vi "IO test DAQ read write.vi"() -> ()   [LabVIEW 2016]
panel:
  in  "Array 3":dbl[](array[numeric])
  in  "Array 2":bool[](array[boolean])
  out "Array":bool[](array[boolean])
  in  "Tab Control":enum32{"Page 1", "Page 2"}(tab)
  in  "write":bool
  in  "Read":bool
  in  "stop":bool
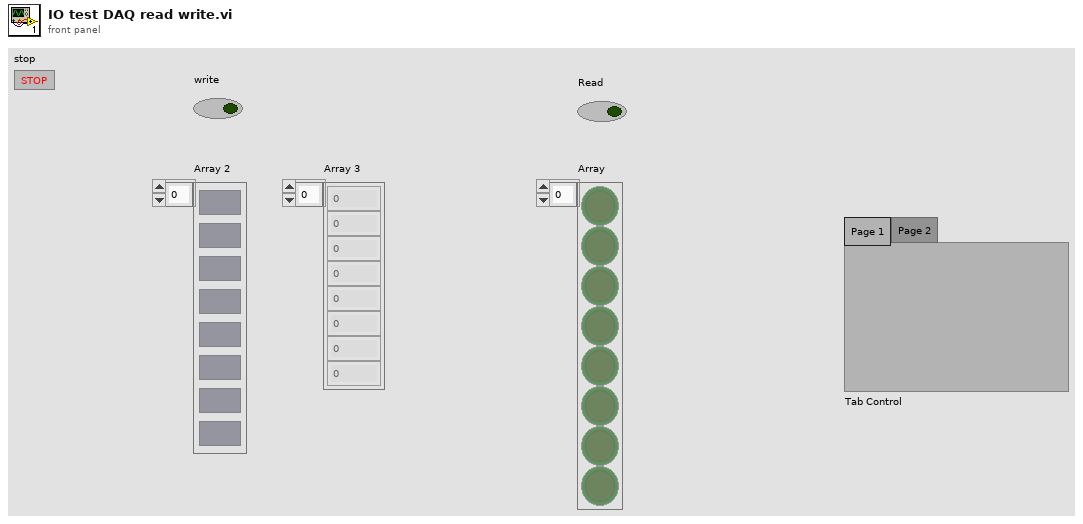
[diagram p1: front panel]
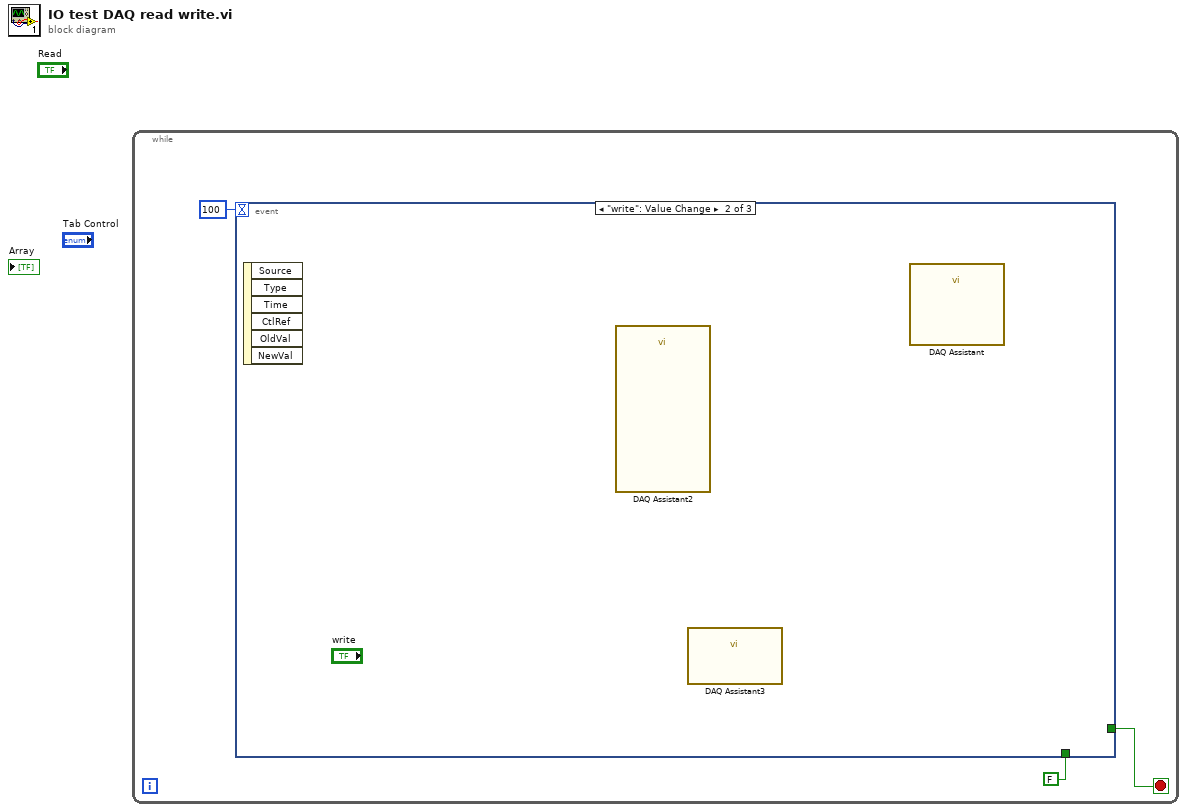
[diagram p0: block diagram]
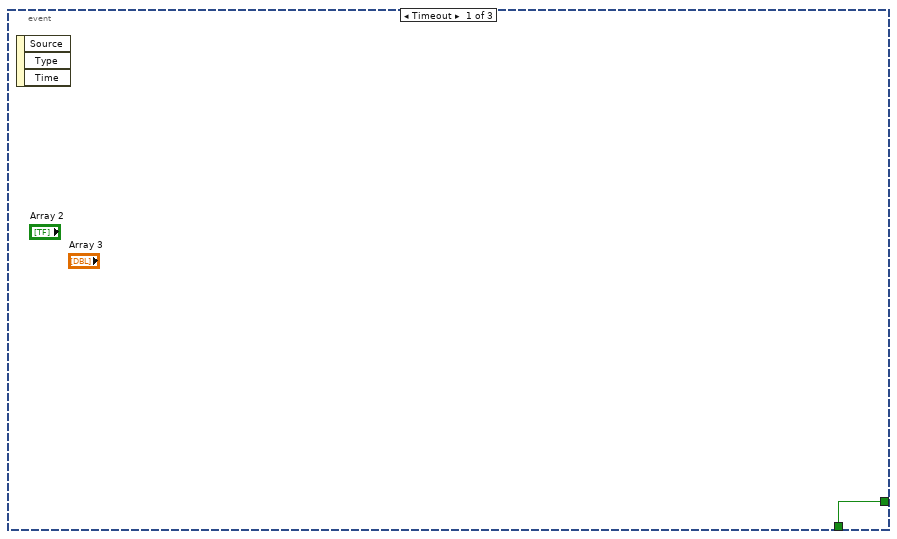
[diagram p2: hidden frame]
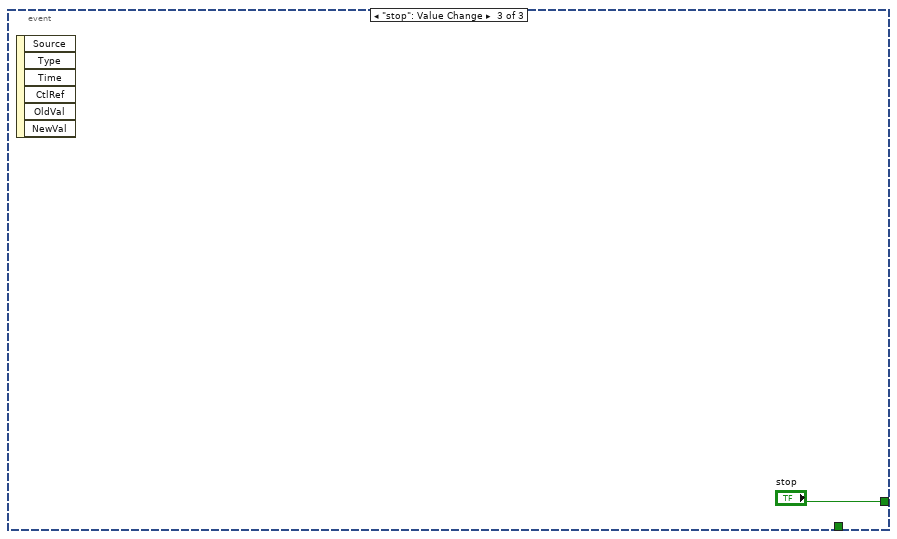
[diagram p3: hidden frame]
diagram:
  n1 = while {
    stop <- w3 stop-if-true
    n2 = event shown="[1] \"write\": Value Change" {
      selector: _ -> [_ _ _]
      dyn-events: _ -> [_ _ _]
      timeout: 100 -> [_ _ _]
      tunnel: [w4 _ "stop"] -> w3
      tunnel: FALSE -> [w4 _ _]
      event Timeout {
        n3 = event-data() -> ()  [unwired: 1 in, 3 out]
      }
      event "write": Value Change {
        n4 = event-data() -> ()  [unwired: 1 in, 6 out]
        n5 = call "DAQ Assistant2"() -> ()  [unwired: 18 in, 2 out]
        n6 = call "DAQ Assistant3"() -> ()  [unwired: 12 in]
        n7 = call "DAQ Assistant"() -> ()  [unwired: 18 in, 2 out]
      }
      event "stop": Value Change {
        n8 = event-data() -> ()  [unwired: 1 in, 6 out]
      }
    }
  }
